vi "OTG Reader and Read Rack Demo.vi"() -> ()   [LabVIEW 2024]
uses:
  <instrlib>/OptoMMP/OptoMMP.lvlib
panel:
  out "Output Data":cluster{"Array out":sgl[]}[](array[cluster])
  out "Loop Time (s)":dbl
  in  "Stop":bool
  out "Error Indicator":errorcluster
  in  "OTG File Path":path
  # "Copyright (c) 2025 California Institute of Technology (Caltech).\nU.S. Government sponsorship acknowledged.\n\nLicensed under the Apache License, Version 2.0 (the \"License\");\nyou may not use this file except in compliance with the License.\nYou may obtain a copy of the License at\n\n    http://www.apache.org/licenses/LICENSE-2.0\n\nUnless required by applicable law or agreed to in writing, software\ndistributed under the License is distributed on an \"AS IS\" BASIS,\nWITHOUT WARRANTIES OR CONDITIONS OF ANY KIND, either express or implied.\nSee the License for the specific language governing permissions and\nlimitations under the License."
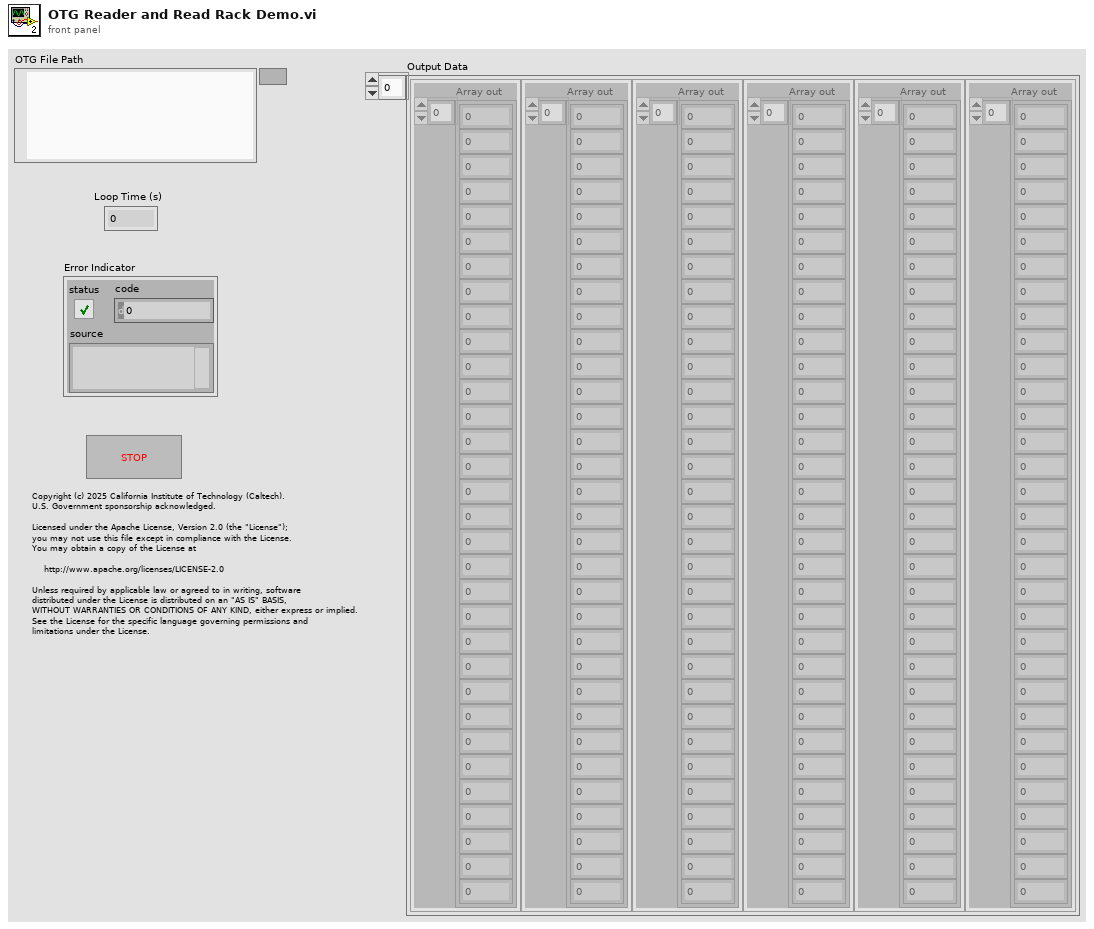
[diagram p1: front panel]
types:
  T1 = cluster{"Points":i32[], "Point Types":string[], "IP address":string}[]
  T2 = cluster{"Points":i32[], "Point Types":string[], "IP address":string, "Connection ID":refnum<k5>}
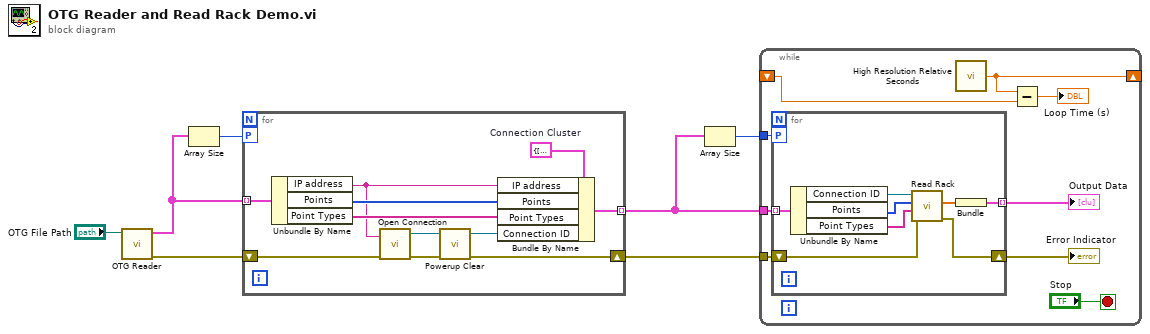
[diagram p0: block diagram]
diagram:
  n1 = call <instrlib>:"OTG Reader.vi"("OTG File Path"="OTG File Path") -> ("Read Spreadsheet Error"=w5:errorcluster, "Opto 22 Rack Array"=w6:T1)  [unwired: 9 in]
  n2 = Array Size(array=w6) -> (size(s)=w4:i32)
  n3 = for {
    tunnel: w6 -> [w16] mode=indexing
    workers-P: w4 -> [_]
    tunnel: [w13] -> w2 mode=indexing
    shift-right: [w8] -> w1
    shift-left: w5 -> [w9]
    w15 = T2 {"Points"=[], "Point Types"=[], "IP address"="", "Connection ID"=refnum}  # Connection Cluster
    n4 = Unbundle By Name(w16) -> ("IP address"=w10:string, "Points"=w12:i32[], "Point Types"=w11:string[])
    n5 = call <instrlib>:"Open Connection.vi"("error in (no error)"=w9, "Client IP Address"=w10) -> ("error out"=w17:errorcluster, "TCP Network Connection out"=w18:refnum<k5>)  [unwired: 8 in]
    n6 = call <instrlib>:"Powerup Clear.vi"("error in (no error)"=w17, "TCP Network Connection in"=w18) -> ("error out"=w8:errorcluster, "connection ID out"=w14:refnum<k5>)  [unwired: 8 in]
    n7 = Bundle By Name(cluster=w15, "IP address"=w10, "Points"=w12, "Point Types"=w11, "Connection ID"=w14) -> (w13:T2)
  }
  n8 = Array Size(array=w2) -> (size(s)=w3:i32)
  n9 = while {
    tunnel: w3 -> [w27]
    tunnel: w2 -> [w26]
    tunnel: w1 -> [w25]
    shift-right: [w22] -> _
    shift-left: _ -> [w21]
    stop <- "Stop" stop-if-true
    n10 = for {
      tunnel: w26 -> [w32] mode=indexing
      shift-right: [w30] -> w24
      shift-left: w25 -> [w31]
      workers-P: w27 -> [_]
      tunnel: [w28] -> w19 mode=indexing
      n11 = Unbundle By Name(w32) -> ("Connection ID"=w35:refnum<k5>, "Points"=w33:i32[], "Point Types"=w34:string[])
      n12 = call <instrlib>:"Read Rack.vi"("error in (no error)"=w31, "Point Types"=w34, "Points"=w33, "TCP Network Connection in"=w35) -> ("error out"=w30:errorcluster, "Array out"=w29:sgl[])  [unwired: 5 in, 1 out]
      n13 = Bundle("Array out"=w29) -> (w28:cluster{"Array out":sgl[]})  [unwired: 1 in]
    }
    "Error Indicator" <- w24
    "Output Data" <- w19
    n14 = call <vilib>:"High Resolution Relative Seconds.vi"() -> ("relative seconds"=w22:dbl)
    n15 = Subtract(x=w22, y=w21) -> (x-y=→"Loop Time (s)":dbl)
  }
